vi "Dialog_Configure Tiling.vi"(9 "Index of Tiling":i32, 10 "Tbl Refnum":refnum<vi>, 11 "Tree Refnum":refnum<vi>) -> (1 "Empty Array/Cancelled?":bool, 2 "Index of 2DFrame.Scan":i32, 3 "Updated Macro String Array":string[](array[string]), 4 "Skip configure 2D settings?":bool)   [LabVIEW 2012]
doc: "SciScan 1.2 160622"
uses:
  Z-Scan Types.ctl
  Custom Controls/scan mode main settings tab.ctl
  FGV_MacroCore_Commands.ctl
  Create Preset commands ENUM.ctl
  GFG/GFGnumericGet.vi
  GFG/GFGfpRefGet.vi
  GFG/GFG library.lvlib
panel:
  out "bottom/right abs":cluster{"abs x":dbl, "abs y":dbl, "abs z":dbl}
  out "bottom/right rel":cluster{"rel x":dbl, "rel y":dbl, "rel z":dbl}
  out "top/left rel":cluster{"rel x":dbl, "rel y":dbl, "rel z":dbl}
  out "top/left abs":cluster{"abs x":dbl, "abs y":dbl, "abs z":dbl}
  in  "Add Bottom/Right Pos":bool
  in  "Add Top/Left Pos":bool
  in  "Cancel Button":bool
  in  "Tiling Type":T1=enum."Slow Z"
  in  "Overlap %":dbl=20.0 min=-100.0 max=100.0
  in  "Frames Per Tile":dbl caption="Frames/Tile" min=4.0 step=4.0
  in  "OK Button":bool
  out "error out":errorcluster
  in  "error in (no error)":errorcluster
  # "You have selected the Tiling Preset \nThe Macro for carrying out the Tiling will be auto-generated for you\nbased on your configuration"
  # "Please note that stitching of tiled images is not supported"
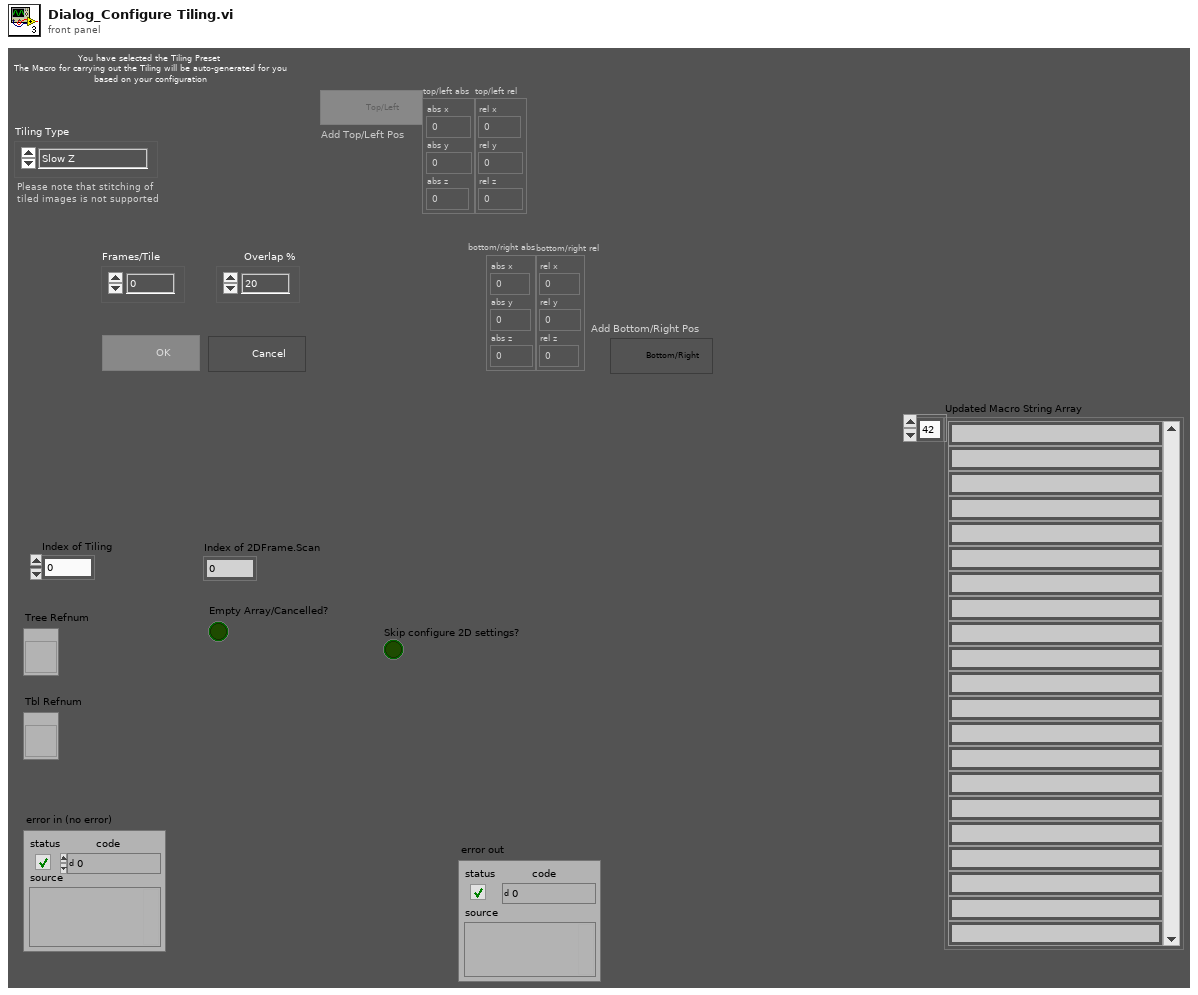
[diagram p1: front panel]
types:
  T1 = typedef "Z-Scan Types.ctl" = enum16{"Single Plane", "Slow Z", "Z-Stack (Regular)", "Fast Z (Piezo)"}
  T2 = typedef "scan mode main settings tab.ctl" = enum32{"2D frame", "2D line scan", "general settings", "Z Stack", "piezo"}
  T3 = cluster{"OK Button":refnum<vi>, "Add Top/Left Pos":refnum<vi>, "Add Bottom/Right Pos":refnum<vi>}
  T4 = enum8{"Enabled", "Disabled", "Disabled and Grayed Out"}
  T5 = typedef "FGV_MacroCore_Commands.ctl" = enum16{"Initialize", "Get Array", "Load macro from file", "Insert Item", "Insert at End", "Edit Parameter String", "Delete instruction", "Move Items", "Save", "SaveAs", "UpdateInfoTable", "Edit Settings File", "New Macro", "Read Temp File", "Delete Multiple"}
  T6 = cluster{"Left Cell String":string, "Child Text":string[], "Child Tag":string, "Item Indent":i32, "Child Only?":bool, "Glyph Index":i32}
  T7 = typedef "Create Preset commands ENUM.ctl" = enum16{"Slow.Z_Move.To.Pos", "Slow.Z_Laser.Power", "Slow.Z_Record", "Tiling_Move.To.Pos", "Tiling_Laser.Power", "Tiling_Record"}
  T8 = cluster{"Left Cell String":string, "Child Text":string[], "Child Tag":string, "Item Indent":i32, "Child Only?":bool, "Glyph Index":i32}[]
  T9 = cluster{"WaveformChartRef":refnum<vi>, "DigitalRef":refnum<vi>, "ArrayRef":refnum<vi>, "TabControlRef":refnum<vi>, "EnumRef":refnum<vi>, "RingRef":refnum<vi>, "BooleanRef":refnum<vi>, "KnobRef":refnum<vi>, "SlideRef":refnum<vi>, "PathRef":refnum<vi>, "StringRef":refnum<vi>, "ComboBox":refnum<vi>, "WaveformGraphRef":refnum<vi>}
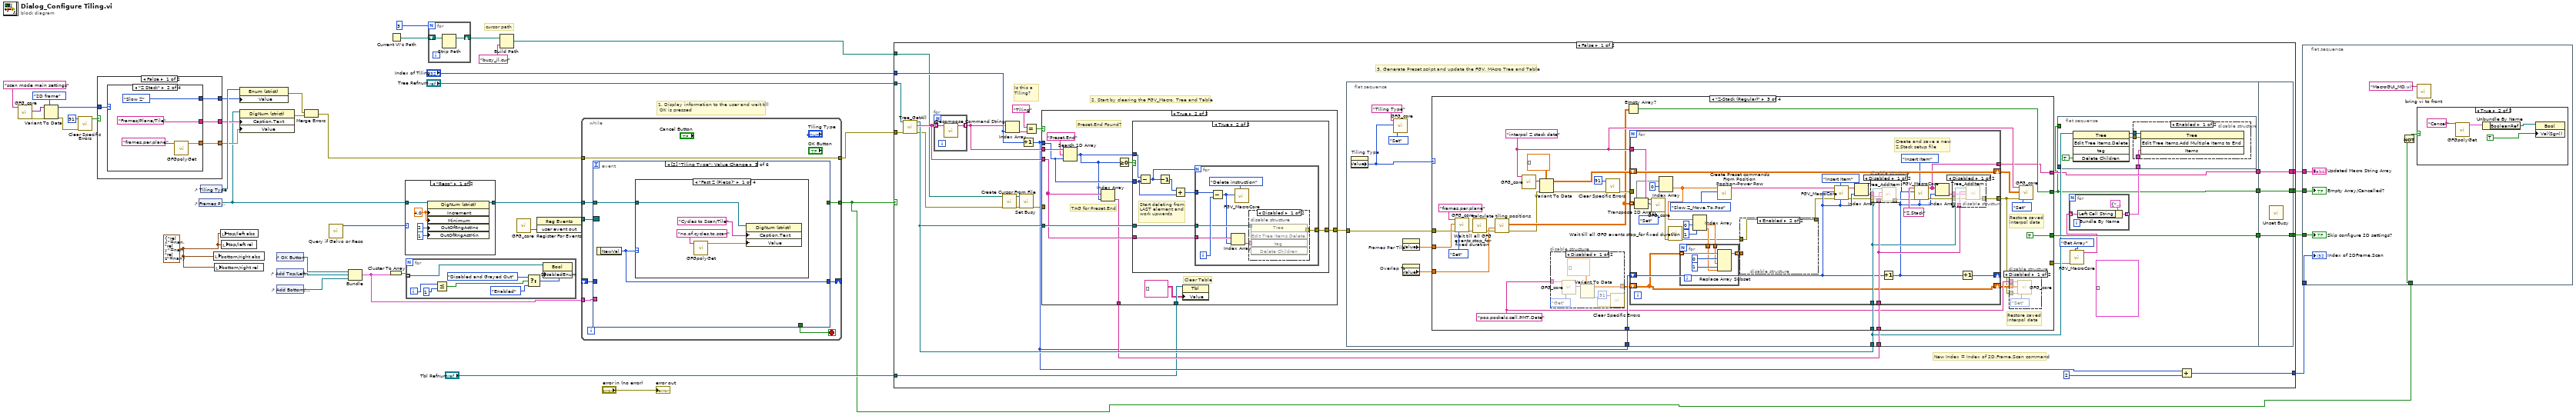
[diagram p0: block diagram]
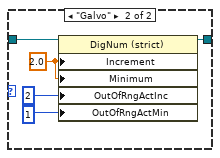
[diagram p3: hidden frame]
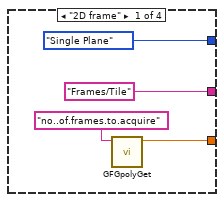
[diagram p4: hidden frame]
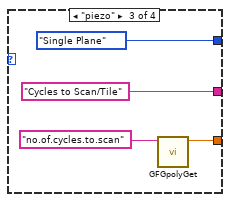
[diagram p5: hidden frame]
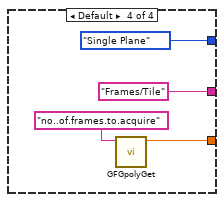
[diagram p6: hidden frame]
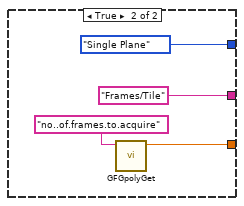
[diagram p7: hidden frame]
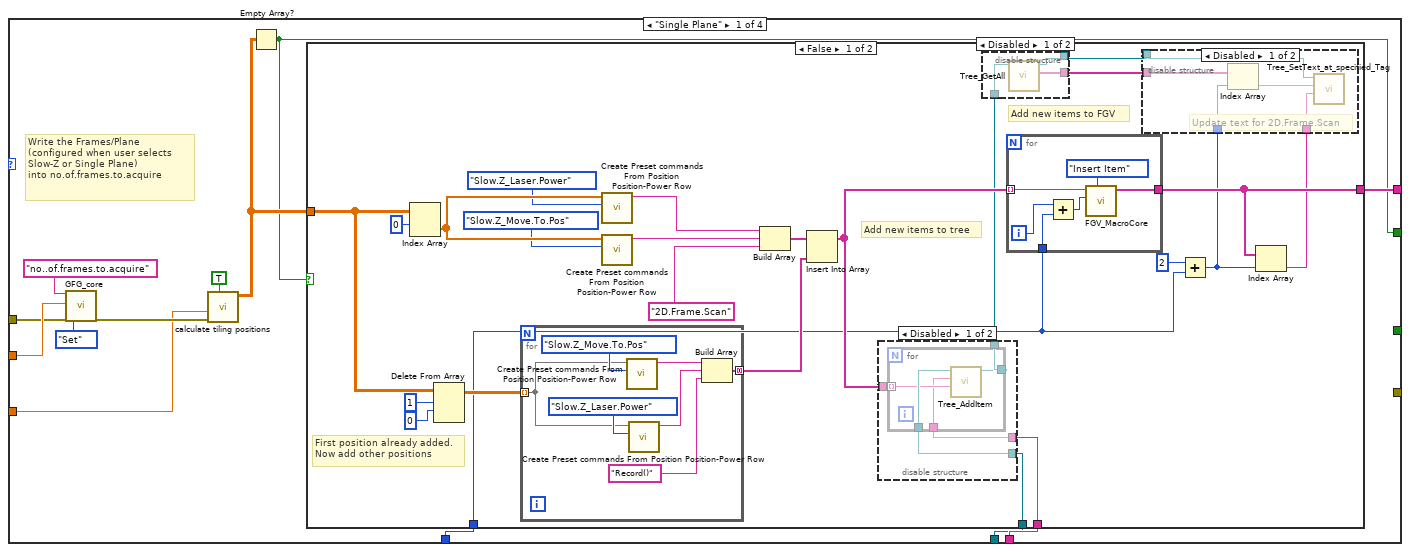
[diagram p9: hidden frame]
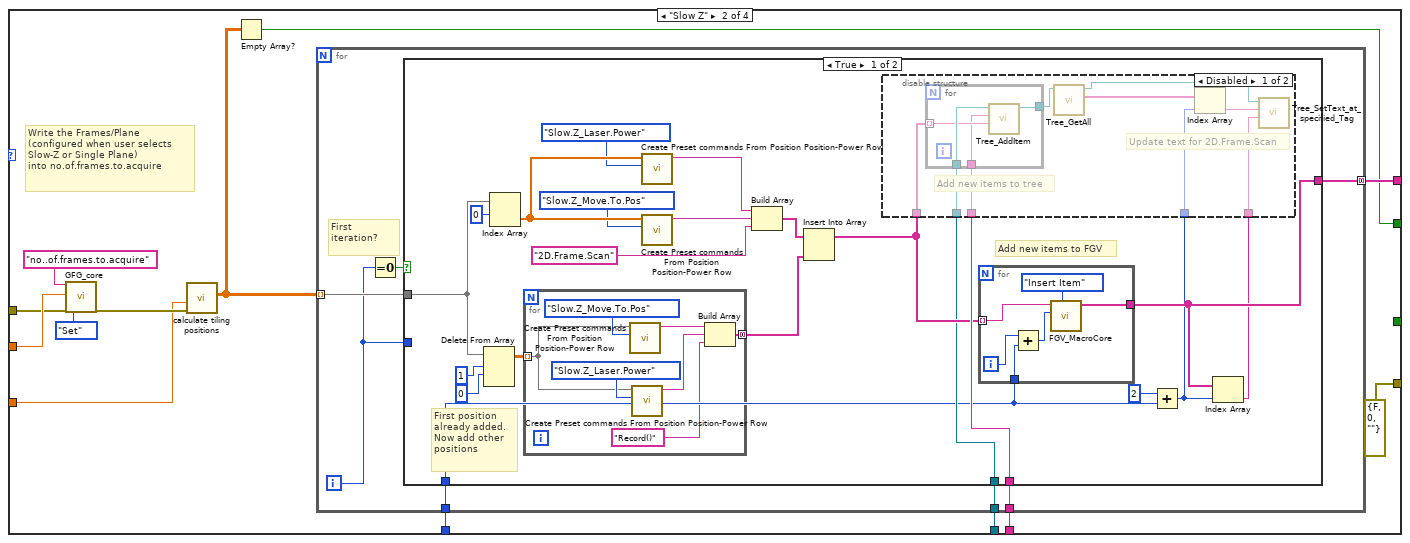
[diagram p14: hidden frame]
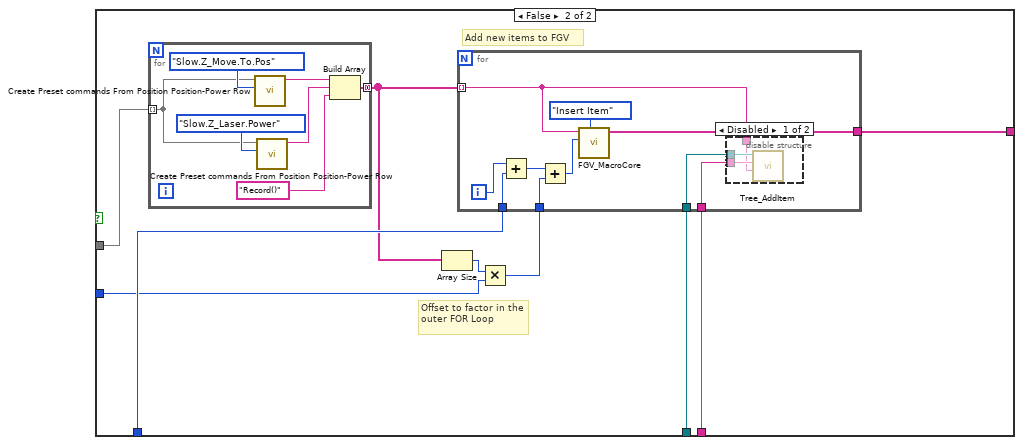
[diagram p16: hidden frame]
diagram:
  w1 = cluster{"rel x":dbl, "rel y":dbl, "rel z":dbl} {"rel x"=nan, "rel y"=nan, "rel z"=nan} ("rel pos out")
  # "1. Display information to the user and wait till\n OK is pressed"
  # "cursor path"
  n1 = call "GFG_core.vi"("Variable Name in"="scan mode main settings") -> ("Variant Out"=w23:variant, "error out"=w22:errorcluster)  [unwired: 12 in, 5 out]
  n2 = Variant To Data(error in=w22, type=scan_mode_main_settings_tab."2D frame" ("scan mode main settings"), Variant=w23) -> (data=w18:T2, error out=w20:errorcluster)
  n3 = call "Clear Specific Errors.vi"("Error In"=w20, "Error number In"=91) -> ("Error Cleared?"=w19:bool)  [unwired: 8 in, 1 out]
  n4 = case shown="False" w19 {
    tunnel: w18 -> [w45 _]
    tunnel: [w44 Z-Scan_Types."Single Plane" ("Value")] -> w16
    tunnel: [w43 "Frames/Tile" ("Caption.Text")] -> w15
    tunnel: [w42 w62] -> w14
    frame False {
      n5 = case shown="\"Z Stack\"" w45 {
        tunnel: [Z-Scan_Types."Single Plane" ("Value") Z-Scan_Types."Slow Z" ("Value") Z-Scan_Types."Single Plane" ("Value") Z-Scan_Types."Single Plane" ("Value")] -> w44
        tunnel: ["Frames/Tile" ("Caption.Text") "Frames/Plane/Tile" ("Caption.Text") "Cycles to Scan/Tile" ("Caption.Text") "Frames/Tile" ("Caption.Text")] -> w43
        tunnel: [w46 w52 w56 w58] -> w42
        frame "2D frame" {
          n6 = call-poly "GFGpolyGet.vi"("Variable Name in"="no..of.frames.to.acquire") -> ("Numeric"=w46:dbl)  [unwired: 8 in, 2 out]
        }
        frame "Z Stack" {
          n7 = call-poly "GFGpolyGet.vi"("Variable Name in"="frames.per.plane") -> ("Numeric"=w52:dbl)  [unwired: 8 in, 2 out]
        }
        frame "piezo" {
          n8 = call-poly "GFGpolyGet.vi"("Variable Name in"="no.of.cycles.to.scan") -> ("Numeric"=w56:dbl)  [unwired: 8 in, 2 out]
        }
        frame Default {
          n9 = call-poly "GFGpolyGet.vi"("Variable Name in"="no..of.frames.to.acquire") -> ("Numeric"=w58:dbl)  [unwired: 8 in, 2 out]
        }
      }
    }
    frame True {
      n10 = call-poly "GFGpolyGet.vi"("Variable Name in"="no..of.frames.to.acquire") -> ("Numeric"=w62:dbl)  [unwired: 8 in, 2 out]
    }
  }
  n11 = control-ref of="Frames Per Tile"() -> (w9:refnum<vi>)
  n12 = control-ref of="Tiling Type"() -> (w17:refnum<vi>)
  n13 = local write "bottom/right abs"(w1) -> ()
  n14 = local write "bottom/right rel"(w1) -> ()
  n15 = local write "top/left abs"(w1) -> ()
  n16 = local write "top/left rel"(w1) -> ()
  n17 = property class="Enum (strict)"(reference=w17, "Value"=w16) -> (error out=w13:errorcluster)  [unwired: 1 in, 1 out]
  n18 = property class="DigNum (strict)"(reference=w9, "Caption.Text"=w15, "Value"=w14) -> (error out=w12:errorcluster)  [unwired: 1 in, 1 out]
  n19 = control-ref of="OK Button"() -> (w7:refnum<vi>)
  n20 = control-ref of="Add Top/Left Pos"() -> (w6:refnum<vi>)
  n21 = control-ref of="Add Bottom/Right Pos"() -> (w5:refnum<vi>)
  n22 = Merge Errors(w13, w12) -> (w11:errorcluster)
  n23 = call "Query if Galvo or Reso.vi"() -> ("System Type"=w10:enum16{"Galvo", "Reso"})  [unwired: 10 in, 1 out]
  n24 = Bundle("OK Button"=w7, "Add Top/Left Pos"=w6, "Add Bottom/Right Pos"=w5) -> (w3:T3)  [unwired: 1 in]
  n25 = Cluster To Array(cluster=w3) -> (array=w4:refnum<vi>[])
  n26 = Current VI's Path() -> (path=w35:path)
  n27 = case shown="\"Reso\"" w10 {
    tunnel: w9 -> [w70 w75]
    tunnel: [w67 w72] -> w8
    frame "Reso" {
      w69 = 4.0 ("Data Entry Limits:Increment")
      n28 = property class="DigNum (strict)"(reference=w70, "Increment"=w69, "Minimum"=w69, "OutOfRngActInc"=u8 2 ("Response to Value Outside Limits:Minimum"), "OutOfRngActMin"=u8 1 ("Response to Value Outside Limits:Minimum")) -> (reference out=w67:refnum<vi>)  [unwired: 1 in, 1 out]
    }
    frame "Galvo" {
      w74 = 2.0 ("Data Entry Limits:Increment")
      n29 = property class="DigNum (strict)"(reference=w75, "Increment"=w74, "Minimum"=w74, "OutOfRngActInc"=u8 2 ("Response to Value Outside Limits:Minimum"), "OutOfRngActMin"=u8 1 ("Response to Value Outside Limits:Minimum")) -> (reference out=w72:refnum<vi>)  [unwired: 1 in, 1 out]
    }
  }
  n30 = for {
    tunnel: w4 -> [w82] mode=indexing
    i -> [w81]
    n31 = Less Or Equal?(x=w81, y=1) -> (x <= y?=w77:bool)
    n32 = Select(t=T4."Disabled and Grayed Out" ("Disabled"), s=w77, f=T4."Enabled" ("Disabled")) -> (s? t:f=w76:T4)
    n33 = property class="Bool"(reference=w82, "DisabledEnum"=w76) -> ()  [unwired: 1 in, 2 out]
  }
  n34 = for {
    N: 3 -> [_]
    shift-right: [w83] -> w34
    shift-left: w35 -> [w84]
    n35 = Strip Path(path=w84) -> (stripped path=w83:path)  [unwired: 1 out]
  }
  n36 = Build Path(base path=w34, name or relative path="busy_il.cur") -> (appended path=w28:path)
  n37 = call "GFG_core.vi"() -> ("user event out"=w41:refnum<user-event>)  [unwired: 13 in, 6 out]
  n38 = register-events(w41) -> (reference out=w40:refnum<event-registration>)  [unwired: 2 in, 1 out]
  n39 = while {
    tunnel: w40 -> [w92]
    tunnel: w11 -> [w90]
    tunnel: [w90] -> w26
    tunnel: [w89] -> w2
    tunnel: w8 -> [w88]
    shift-right: [w87] -> _
    shift-left: _ -> [w86]
    tunnel: w3 -> [w85]
    stop <- w91 stop-if-true
    n40 = event shown="[2] \"Tiling Type\": Value Change" {
      selector: w92 -> [_ _ _ _ _ _]
      dyn-events: _ -> [_ _ _ _ _ _]
      timeout: _ -> [_ _ _ _ _ _]
      tunnel: [TRUE w102 _ _ _ w142] -> w91
      tunnel: [_ _ _ _ _ w142] -> w89
      tunnel: w88 -> [_ _ w106 _ _ _]
      tunnel: [w99 w101 w105 w132 w140 w141] -> w87
      tunnel: w86 -> [w99 w101 _ w132 w140 w141]
      tunnel: w85 -> [_ _ _ w127 w134 _]
      event "OK Button": Value Change {
        n41 = event-data() -> ()  [unwired: 1 in, 1 out]
        n42 = call "GFG_core.vi"("Variable Name in"="Frames Per Tile", "Variant in"="Frames Per Tile", "Action"=enum16{"Init", "Set", "Get", "Clear"}."Set") -> ()  [unwired: 10 in, 7 out]
        n43 = call "GFG_core.vi"("Variable Name in"="Overlap", "Variant in"="Overlap %", "Action"=enum16{"Init", "Set", "Get", "Clear"}."Set") -> ()  [unwired: 10 in, 7 out]
      }
      event User Event {
        n44 = event-data() -> ("Variable Name"=w103:string)  [unwired: 1 in]
        n45 = case shown="\"QUIT\"" w103 {
          tunnel: [_ TRUE] -> w102
          frame "False", Default {
          }
          frame "QUIT" {
          }
        }
      }
      event Value Change {
        n46 = event-data() -> ("NewVal"=w105:T1)  [unwired: 1 in]
        n47 = case shown="\"Fast Z (Piezo)\"" w105 {
          tunnel: w106 -> [w108 w112 w117 w121]
          frame "Fast Z (Piezo)" {
            n48 = call-poly "GFGpolyGet.vi"("Variable Name in"="no.of.cycles.to.scan") -> ("Numeric"=w107:dbl)  [unwired: 8 in, 2 out]
            n49 = property class="DigNum (strict)"(reference=w108, "Caption.Text"="Cycles to Scan/Tile", "Value"=w107) -> ()  [unwired: 1 in, 2 out]
          }
          frame "Slow Z" {
            n50 = call-poly "GFGpolyGet.vi"("Variable Name in"="frames.per.plane") -> ("Numeric"=w111:dbl)  [unwired: 8 in, 2 out]
            n51 = property class="DigNum (strict)"(reference=w112, "Caption.Text"="Frames/Plane/Tile", "Value"=w111) -> ()  [unwired: 1 in, 2 out]
          }
          frame "Z-Stack (Regular)" {
            n52 = call-poly "GFGpolyGet.vi"("Variable Name in"="frames.per.plane") -> ("Numeric"=w116:dbl)  [unwired: 8 in, 2 out]
            n53 = property class="DigNum (strict)"(reference=w117, "Caption.Text"="Frames/Plane/Tile", "Value"=w116) -> ()  [unwired: 1 in, 2 out]
          }
          frame "Single Plane" {
            n54 = call-poly "GFGpolyGet.vi"("Variable Name in"="no..of.frames.to.acquire") -> ("Numeric"=w119:dbl)  [unwired: 8 in, 2 out]
            n55 = property class="DigNum (strict)"(reference=w121, "Caption.Text"="Frames/Tile", "Value"=w119) -> ()  [unwired: 1 in, 2 out]
          }
        }
      }
      event "Add Top/Left Pos": Value Change {
        n56 = event-data() -> ()  [unwired: 1 in, 1 out]
        n57 = Unbundle By Name(w127) -> ("Add Bottom/Right Pos"=w125:refnum<vi>, "OK Button"=w123:refnum<vi>)
        n58 = call "current abs pos to rel pos.vi"() -> ("rel pos out"=w128:cluster{"rel x":dbl, "rel y":dbl, "rel z":dbl}, "abs pos out"=→"top/left abs":cluster{"abs x":dbl, "abs y":dbl, "abs z":dbl})  [unwired: 10 in]
        "top/left rel" <- w128
        n59 = property class="Bool"(reference=w125, "DisabledEnum"=T4."Disabled and Grayed Out" ("Disabled")) -> ()  [unwired: 1 in, 2 out]
        n60 = property class="Bool"(reference=w123, "DisabledEnum"=T4."Enabled" ("Disabled")) -> ()  [unwired: 1 in, 2 out]
        n61 = call "GFG_core.vi"("Variable Name in"="top left tile pos", "Variant in"=w128, "Action"=enum16{"Init", "Set", "Get", "Clear"}."Set") -> ()  [unwired: 10 in, 7 out]
      }
      event "Add Bottom/Right Pos": Value Change {
        n62 = event-data() -> ()  [unwired: 1 in, 1 out]
        n63 = Unbundle By Name(w134) -> ("Add Top/Left Pos"=w133:refnum<vi>)
        n64 = call "current abs pos to rel pos.vi"() -> ("rel pos out"=w137:cluster{"rel x":dbl, "rel y":dbl, "rel z":dbl}, "abs pos out"=→"bottom/right abs":cluster{"abs x":dbl, "abs y":dbl, "abs z":dbl})  [unwired: 10 in]
        "bottom/right rel" <- w137
        n65 = property class="Bool"(reference=w133, "DisabledEnum"=T4."Enabled" ("Disabled")) -> ()  [unwired: 1 in, 2 out]
        n66 = call "GFG_core.vi"("Variable Name in"="bottom right tile pos", "Variant in"=w137, "Action"=enum16{"Init", "Set", "Get", "Clear"}."Set") -> ()  [unwired: 10 in, 7 out]
      }
      event "Cancel Button": Value Change {
        w142 = TRUE
        n67 = event-data() -> ()  [unwired: 1 in, 1 out]
      }
    }
  }
  n68 = case shown="False" w2 {
    selector: w2 -> [_ w577]
    tunnel: "Index of Tiling" -> [w162 _]
    tunnel: "Tree Refnum" -> [w161 _]
    tunnel: [w159 _] -> w36
    tunnel: "Tbl Refnum" -> [w153 _]
    tunnel: [w152 _] -> w30
    tunnel: [w151 w577] -> w29
    tunnel: w28 -> [w148 _]
    tunnel: [w145 _] -> w27
    tunnel: w26 -> [w144 _]
    frame False {
      # "New Index = Index of 2D.Frame.Scan command"
      # "3. Generate Preset script and update the FGV, MAcro Tree and Table"
      # "2. Start by clearing the FGV_Macro, Tree and Table"
      # "Is this a Tiling?"
      n69 = call "Tree_GetAll.vi"("Error In"=w144, "Tree Refnum IN"=w161) -> ("Error Out"=w147:errorcluster, "Tags"=w158:string[], "Tree Refnum OUT"=w156:refnum<vi>)  [unwired: 6 in, 1 out]
      n70 = for {
        tunnel: w158 -> [w546] mode=indexing
        tunnel: [w545] -> w157 mode=indexing
        n71 = call "Decompose Command String.vi"("Command IN"=w546) -> ("Action"=w545:string)  [unwired: 7 in, 3 out]
      }
      n72 = call <vilib>:"Create Cursor From File.vi"("error in (no error)"=w147, "cursor file"=w148) -> ("error out"=w150:errorcluster, "cursor ID"=w149:refnum<k1>)  [unwired: 8 in]
      n73 = Index Array(array=w157, index=w162) -> (element=w165:string)
      n74 = call <vilib>:"Set Busy.vi"("error in (no error)"=w150, "cursor ID"=w149) -> ("error out"=w146:errorcluster)  [unwired: 8 in, 1 out]
      n75 = Increment(x=w162) -> (x+1=w154:i32)
      n76 = Equal?(x="Tiling" ("Variable Name in"), y=w165) -> (x = y?=w163:bool)
      n77 = case shown="True" w163 {
        tunnel: w158 -> [_ w553]
        tunnel: w157 -> [_ w557]
        tunnel: w154 -> [_ w551]
        tunnel: w156 -> [_ w555]
        tunnel: [_ w554] -> w143
        tunnel: [_ w550] -> w155
        tunnel: w153 -> [_ w548]
        tunnel: w146 -> [_ _]
        frame False {
        }
        frame True {
          # "Clear Table"
          # "TAG for Preset.End"
          # "Preset.End Found?"
          n78 = Search 1D Array(1D array=w557, element="Preset.End", start index (0)=w551) -> (index of element=w549:i32)
          n79 = Index Array(array=w553, index=w549) -> (element=w550:string)
          n80 = Greater Or Equal To 0?(x=w549) -> (x >= 0?=w552:bool)
          n81 = case shown="True" w552 {
            tunnel: w549 -> [_ w565]
            tunnel: w555 -> [_ w561]
            tunnel: [_ w560] -> w554
            tunnel: w551 -> [_ w559]
            tunnel: w553 -> [_ w558]
            frame False {
            }
            frame True {
              # "Start deleting from LAST element and work upwards"
              n82 = Subtract(x=w565, y=w559) -> (x-y=w564:i32)
              n83 = Decrement(x=w564) -> (x-1=w563:i32)
              n84 = Add(x=w563, y=w559) -> (x+y=w562:i32)
              n85 = for {
                N: w564 -> [_]
                tunnel: w562 -> [w571]
                tunnel: w561 -> [w570]
                tunnel: w558 -> [w569]
                tunnel: [w566] -> w560
                i -> [w572]
                n86 = Subtract(x=w571, y=w572) -> (x-y=w568:i32)
                n87 = Index Array(array=w569, index=w568) -> (element=w567:string)
                n88 = call "FGV_MacroCore.vi"("MacroFGV_Commands"=FGV_MacroCore_Commands."Delete instruction", "Start Index"=w568) -> ()  [unwired: 5 in, 5 out]
                n89 = disable-structure shown="Disabled" {
                  disable-tunnel: w570 -> [w576 _]
                  disable-tunnel: w567 -> [w575 _]
                  disable-tunnel: [w574 _] -> w566
                  frame Disabled {
                    n90 = invoke class="Tree" method="Edit Tree Items.Delete"(reference=w576, "tag"=w575) -> (error out=w574:errorcluster)  [unwired: 3 in, 4 out]
                  }
                  frame Enabled {
                  }
                }
              }
            }
          }
          n91 = property class="Tbl"(reference=w548, "Value"=string[][] []) -> ()  [unwired: 1 in, 2 out]
        }
      }
      n92 = flat-sequence {
        tunnel: w156 -> [w178]
        tunnel: w155 -> [w184]
        tunnel: w154 -> [w183]
        tunnel: [w177] -> w168
        tunnel: [w175] -> w167
        tunnel: [w181] -> w166
        tunnel: w143 -> [w182]
        tunnel: [w543] -> w151
        tunnel: [w544] -> w152
        tunnel: w168 -> [w544]
        tunnel: w167 -> [w543]
        tunnel: [w542] -> w145
        tunnel: w166 -> [w542]
        frame #0 {
          (unwired) T8 [] ("Items")
          n93 = property on="Tiling Type" class="Enum (strict)"() -> ("Value"=w169:T1)  [unwired: 2 in, 2 out]
          n94 = call "GFG_core.vi"("Variable Name in"="Tiling Type", "Variant in"=w169, "Action"=enum16{"Init", "Set", "Get", "Clear"}."Set") -> ()  [unwired: 10 in, 7 out]
          n95 = property on="Frames Per Tile" class="DigNum (strict)"() -> ("Value"=w180:dbl)  [unwired: 2 in, 2 out]
          n96 = property on="Overlap %" class="DigNum (strict)"() -> ("Value"=w179:dbl)  [unwired: 2 in, 2 out]
          n97 = case shown="\"Z-Stack (Regular)\"" w169 {
            tunnel: w178 -> [w207 w273 w373 w477]
            tunnel: w184 -> [w208 w274 w372 w476]
            tunnel: w183 -> [w206 w272 w377 w481]
            tunnel: [w205 w271 w371 w475] -> w177
            tunnel: [w196 w264 w384 w488] -> w175
            tunnel: w182 -> [w201 w267 w365 w460]
            tunnel: [_ _ TRUE TRUE] -> w181
            tunnel: w180 -> [w204 w270 w361 w459]
            tunnel: w179 -> [w199 w265 w358 w457]
            tunnel: [_ errorcluster {"status"=FALSE, "code"=0, "source"=""} ("error in (no error)") _ _] -> w172
            frame "Single Plane" {
              # "Write the Frames/Plane\n(configured when user selects Slow-Z or Single Plane)\ninto no.of.frames.to.acquire"
              n98 = call "GFG_core.vi"("Variable Name in"="no..of.frames.to.acquire", "Variant in"=w204, "error in (no error)"=w201, "Action"=enum16{"Init", "Set", "Get", "Clear"}."Set") -> ("error out"=w200:errorcluster)  [unwired: 9 in, 6 out]
              n99 = call "calculate tiling positions.vi"("Single Plane?"=TRUE, "error in (no error)"=w200, "overlap percentage"=w199) -> ("2D Array for single plane tiling or Slow Z Tiling"=w198:dbl[][])  [unwired: 6 in, 2 out]
              n100 = Empty Array?(array=w198) -> (empty?=w196:bool)
              n101 = case shown="False" w196 {
                tunnel: w208 -> [w222 _]
                tunnel: w207 -> [w218 _]
                tunnel: w206 -> [w216 _]
                tunnel: [w214 _] -> w205
                tunnel: w198 -> [w209 _]
                frame False {
                  # "Add new items to FGV"
                  # "Add new items to tree"
                  # "First position already added.\nNow add other positions"
                  n102 = Index Array(array=w209, index (row)=0) -> (element=w225:dbl[])  [unwired: 1 in]
                  n103 = Delete From Array(array=w209, length=1, index (row)=0) -> (array with subset deleted=w230:dbl[][])  [unwired: 1 in, 1 out]
                  n104 = for {
                    tunnel: w230 -> [w252] mode=indexing
                    tunnel: [w255] -> w227 mode=concatenating
                    n105 = call "Create Preset commands From Position Position-Power Row.vi"("Create SlowZ commands_Enum"=Create_Preset_commands_ENUM."Slow.Z_Move.To.Pos", "Position-Power Row"=w252) -> ("concatenated string"=w251:string)  [unwired: 9 in]
                    n106 = call "Create Preset commands From Position Position-Power Row.vi"("Create SlowZ commands_Enum"=Create_Preset_commands_ENUM."Slow.Z_Laser.Power", "Position-Power Row"=w252) -> ("concatenated string"=w250:string)  [unwired: 9 in]
                    n107 = Build Array(w251, w250, "Record()" ("Variable Name in")) -> (w255:string[])
                  }
                  n108 = call "Create Preset commands From Position Position-Power Row.vi"("Create SlowZ commands_Enum"=Create_Preset_commands_ENUM."Slow.Z_Laser.Power", "Position-Power Row"=w225) -> ("concatenated string"=w219:string)  [unwired: 9 in]
                  n109 = call "Create Preset commands From Position Position-Power Row.vi"("Create SlowZ commands_Enum"=Create_Preset_commands_ENUM."Slow.Z_Move.To.Pos", "Position-Power Row"=w225) -> ("concatenated string"=w220:string)  [unwired: 9 in]
                  n110 = Build Array(w219, w220, "2D.Frame.Scan" ("Variable Name in")) -> (w228:string[])
                  n111 = Insert Into Array(array=w228, new element=w227) -> (w221:string[])  [unwired: 1 in]
                  n112 = disable-structure shown="Disabled" {
                    disable-tunnel: w222 -> [w239 _]
                    disable-tunnel: w221 -> [w238 _]
                    disable-tunnel: w218 -> [w237 _]
                    disable-tunnel: [w236 _] -> w217
                    frame Disabled {
                      n113 = for {
                        tunnel: w238 -> [w242] mode=indexing
                        tunnel: w237 -> [w243]
                        tunnel: w239 -> [w241]
                        tunnel: [w240] -> w236
                        n114 = call "Tree_AddItem.vi"("NEW String"=w242, "Tag at add position"=w241, "Tree Refnum"=w243) -> ("Tree Refnum OUT"=w240:refnum<vi>)  [unwired: 6 in, 2 out]
                      }
                    }
                    frame Enabled {
                    }
                  }
                  n115 = disable-structure shown="Disabled" {
                    disable-tunnel: w217 -> [w235 _]
                    disable-tunnel: [w234 _] -> w213
                    disable-tunnel: [w233 _] -> w211
                    frame Disabled {
                      n116 = call "Tree_GetAll.vi"("Tree Refnum IN"=w235) -> ("Tags"=w234:string[], "Tree Refnum OUT"=w233:refnum<vi>)  [unwired: 7 in, 2 out]
                    }
                    frame Enabled {
                    }
                  }
                  n117 = for {
                    tunnel: w221 -> [w248] mode=indexing
                    tunnel: [w245] -> w214
                    tunnel: w216 -> [w246]
                    i -> [w247]
                    n118 = Add(x=w247, y=w246) -> (x+y=w244:i32)
                    n119 = call "FGV_MacroCore.vi"("MacroFGV_Commands"=FGV_MacroCore_Commands."Insert Item", "Start Index"=w244, "Macro Command or Info (String)"=w248) -> ("Macro String Array"=w245:string[])  [unwired: 4 in, 4 out]
                  }
                  n120 = Add(x=2 ("y"), y=w216) -> (x+y=w212:i32)
                  n121 = Index Array(array=w214, index=w212) -> (element=w210:string)
                  n122 = disable-structure shown="Disabled" {
                    disable-tunnel: w213 -> [w261 _]
                    disable-tunnel: w212 -> [w260 _]
                    disable-tunnel: w211 -> [w258 _]
                    disable-tunnel: w210 -> [w257 _]
                    frame Disabled {
                      # "Update text for 2D.Frame.Scan"
                      n123 = Index Array(array=w261, index=w260) -> (element=w259:string)
                      n124 = call "Tree_SetText_at_specified_Tag.vi"("New String IN"=w257, "Tag (whose string to be edited)"=w259, "Tree Refnum IN"=w258) -> ()  [unwired: 7 in, 2 out]
                    }
                    frame Enabled {
                    }
                  }
                }
                frame True {
                }
              }
            }
            frame "Slow Z" {
              # "Write the Frames/Plane\n(configured when user selects Slow-Z or Single Plane)\ninto no.of.frames.to.acquire"
              n125 = call "GFG_core.vi"("Variable Name in"="no..of.frames.to.acquire", "Variant in"=w270, "error in (no error)"=w267, "Action"=enum16{"Init", "Set", "Get", "Clear"}."Set") -> ("error out"=w266:errorcluster)  [unwired: 9 in, 6 out]
              n126 = call "calculate tiling positions.vi"("error in (no error)"=w266, "overlap percentage"=w265) -> ("Array 2 - for Zstack tiling use this"=w263:dbl[][][])  [unwired: 7 in, 2 out]
              n127 = Empty Array?(array=w263) -> (empty?=w264:bool)
              n128 = for {
                tunnel: w274 -> [w281]
                tunnel: w273 -> [w280]
                tunnel: w272 -> [w279]
                tunnel: [w278] -> w271 mode=concatenating
                tunnel: w263 -> [w277] mode=indexing
                i -> [w275]
                # "First iteration?"
                n129 = Equal To 0?(x=w275) -> (x = 0?=w276:bool)
                n130 = case shown="True" w276 {
                  tunnel: w281 -> [w293 w330]
                  tunnel: w280 -> [w289 w329]
                  tunnel: w279 -> [w288 w337]
                  tunnel: [w286 w336] -> w278
                  tunnel: w277 -> [w283 w335]
                  tunnel: w275 -> [_ w332]
                  frame True {
                    # "Add new items to FGV"
                    # "First position already added. Now add other positions"
                    n131 = Delete From Array(array=w283, length=1, index (row)=0) -> (array with subset deleted=w300:dbl[][])  [unwired: 1 in, 1 out]
                    n132 = Index Array(array=w283, index (row)=0) -> (element=w296:dbl[])  [unwired: 1 in]
                    n133 = for {
                      tunnel: w300 -> [w324] mode=indexing
                      tunnel: [w327] -> w298 mode=concatenating
                      n134 = call "Create Preset commands From Position Position-Power Row.vi"("Create SlowZ commands_Enum"=Create_Preset_commands_ENUM."Slow.Z_Move.To.Pos", "Position-Power Row"=w324) -> ("concatenated string"=w323:string)  [unwired: 9 in]
                      n135 = call "Create Preset commands From Position Position-Power Row.vi"("Create SlowZ commands_Enum"=Create_Preset_commands_ENUM."Slow.Z_Laser.Power", "Position-Power Row"=w324) -> ("concatenated string"=w322:string)  [unwired: 9 in]
                      n136 = Build Array(w323, w322, "Record()" ("Variable Name in")) -> (w327:string[])
                    }
                    n137 = call "Create Preset commands From Position Position-Power Row.vi"("Create SlowZ commands_Enum"=Create_Preset_commands_ENUM."Slow.Z_Laser.Power", "Position-Power Row"=w296) -> ("concatenated string"=w290:string)  [unwired: 9 in]
                    n138 = call "Create Preset commands From Position Position-Power Row.vi"("Create SlowZ commands_Enum"=Create_Preset_commands_ENUM."Slow.Z_Move.To.Pos", "Position-Power Row"=w296) -> ("concatenated string"=w291:string)  [unwired: 9 in]
                    n139 = Build Array(w290, w291, "2D.Frame.Scan" ("Variable Name in")) -> (w299:string[])
                    n140 = Insert Into Array(array=w299, new element=w298) -> (w292:string[])  [unwired: 1 in]
                    n141 = for {
                      tunnel: w292 -> [w320] mode=indexing
                      tunnel: [w317] -> w286
                      tunnel: w288 -> [w318]
                      i -> [w319]
                      n142 = Add(x=w319, y=w318) -> (x+y=w316:i32)
                      n143 = call "FGV_MacroCore.vi"("MacroFGV_Commands"=FGV_MacroCore_Commands."Insert Item", "Start Index"=w316, "Macro Command or Info (String)"=w320) -> ("Macro String Array"=w317:string[])  [unwired: 4 in, 4 out]
                    }
                    n144 = Add(x=2 ("y"), y=w288) -> (x+y=w285:i32)
                    n145 = Index Array(array=w286, index=w285) -> (element=w284:string)
                    n146 = disable-structure shown="Disabled" {
                      disable-tunnel: w293 -> [w311 _]
                      disable-tunnel: w292 -> [w310 _]
                      disable-tunnel: w289 -> [w309 _]
                      disable-tunnel: w285 -> [w306 _]
                      disable-tunnel: w284 -> [w303 _]
                      frame Disabled {
                        # "Update text for 2D.Frame.Scan"
                        # "Add new items to tree"
                        n147 = for {
                          tunnel: w310 -> [w314] mode=indexing
                          tunnel: w309 -> [w315]
                          tunnel: w311 -> [w313]
                          tunnel: [w312] -> w308
                          n148 = call "Tree_AddItem.vi"("NEW String"=w314, "Tag at add position"=w313, "Tree Refnum"=w315) -> ("Tree Refnum OUT"=w312:refnum<vi>)  [unwired: 6 in, 2 out]
                        }
                        n149 = call "Tree_GetAll.vi"("Tree Refnum IN"=w308) -> ("Tags"=w307:string[], "Tree Refnum OUT"=w304:refnum<vi>)  [unwired: 7 in, 2 out]
                        n150 = Index Array(array=w307, index=w306) -> (element=w305:string)
                        n151 = call "Tree_SetText_at_specified_Tag.vi"("New String IN"=w303, "Tag (whose string to be edited)"=w305, "Tree Refnum IN"=w304) -> ()  [unwired: 7 in, 2 out]
                      }
                      frame Enabled {
                      }
                    }
                  }
                  frame False {
                    # "Offset to factor in the outer FOR Loop"
                    # "Add new items to FGV"
                    n152 = for {
                      tunnel: w335 -> [w353] mode=indexing
                      tunnel: [w356] -> w334 mode=concatenating
                      n153 = call "Create Preset commands From Position Position-Power Row.vi"("Create SlowZ commands_Enum"=Create_Preset_commands_ENUM."Slow.Z_Move.To.Pos", "Position-Power Row"=w353) -> ("concatenated string"=w352:string)  [unwired: 9 in]
                      n154 = call "Create Preset commands From Position Position-Power Row.vi"("Create SlowZ commands_Enum"=Create_Preset_commands_ENUM."Slow.Z_Laser.Power", "Position-Power Row"=w353) -> ("concatenated string"=w351:string)  [unwired: 9 in]
                      n155 = Build Array(w352, w351, "Record()" ("Variable Name in")) -> (w356:string[])
                    }
                    n156 = Array Size(array=w334) -> (size(s)=w333:i32)
                    n157 = Multiply(x=w333, y=w332) -> (x*y=w331:i32)
                    n158 = for {
                      tunnel: w334 -> [w338] mode=indexing
                      tunnel: [w344] -> w336
                      tunnel: w337 -> [w345]
                      tunnel: w331 -> [w342]
                      tunnel: w330 -> [w340]
                      tunnel: w329 -> [w339]
                      i -> [w346]
                      n159 = Add(x=w346, y=w345) -> (x+y=w343:i32)
                      n160 = Add(x=w343, y=w342) -> (x+y=w341:i32)
                      n161 = call "FGV_MacroCore.vi"("MacroFGV_Commands"=FGV_MacroCore_Commands."Insert Item", "Start Index"=w341, "Macro Command or Info (String)"=w338) -> ("Macro String Array"=w344:string[])  [unwired: 4 in, 4 out]
                      n162 = disable-structure shown="Disabled" {
                        disable-tunnel: w340 -> [w350 _]
                        disable-tunnel: w339 -> [w349 _]
                        disable-tunnel: w338 -> [w348 _]
                        frame Disabled {
                          n163 = call "Tree_AddItem.vi"("NEW String"=w348, "Tag at add position"=w350, "Tree Refnum"=w349) -> ()  [unwired: 6 in, 3 out]
                        }
                        frame Enabled {
                        }
                      }
                    }
                  }
                }
              }
            }
            frame "Z-Stack (Regular)" {
              w368 = "pos.pockels.cell.PMT.Data" ("Variable Name in")
              w375 = "interpol Z stack data" ("Variable Name in")
              # "Restore saved \ninterpol data"
              # "Restore saved \ninterpol data"
              n164 = call "GFG_core.vi"("Variable Name in"="frames.per.plane", "Variant in"=w361, "error in (no error)"=w365, "Action"=enum16{"Init", "Set", "Get", "Clear"}."Set") -> ("error out"=w362:errorcluster)  [unwired: 9 in, 6 out]
              n165 = call "Wait till all GFG events stop_for fixed duration.vi"("error in (no error)"=w362) -> ("error out"=w359:errorcluster)  [unwired: 10 in]
              n166 = call "calculate tiling positions.vi"("error in (no error)"=w359, "overlap percentage"=w358) -> ("Array 2 - for Zstack tiling use this"=w360:dbl[][][])  [unwired: 7 in, 2 out]
              n167 = call "GFG_core.vi"("Variable Name in"=w375) -> ("Variant Out"=w383:variant)  [unwired: 12 in, 6 out]
              n168 = Variant To Data(error in=w359, type=dbl[][] [] ("Interpolated Data"), Variant=w383) -> (data=w379:dbl[][], error out=w381:errorcluster)
              n169 = disable-structure shown="Disabled" {
                disable-tunnel: [w390 _] -> w369
                disable-tunnel: w368 -> [w389 _]
                frame Disabled {
                  n170 = call "GFG_core.vi"("Variable Name in"=w389, "Action"=enum16{"Init", "Set", "Get", "Clear"}."Get") -> ("Variant Out"=w391:variant)  [unwired: 11 in, 6 out]
                  n171 = Variant To Data(type=dbl[][] [] ("Interpolated Data"), Variant=w391) -> (data=w390:dbl[][], error out=w393:errorcluster)  [unwired: 1 in]
                  n172 = call "Clear Specific Errors.vi"("Error In"=w393, "Error number In"=91) -> ()  [unwired: 8 in, 2 out]
                }
                frame Enabled {
                }
              }
              n173 = call "Clear Specific Errors.vi"("Error In"=w381, "Error number In"=91) -> ("Error Out"=w378:errorcluster)  [unwired: 8 in, 1 out]
              n174 = Empty Array?(array=w360) -> (empty?=w384:bool)
              n175 = for {
                tunnel: w360 -> [w426] mode=indexing
                shift-right: [w429] -> w374
                shift-left: w379 -> [w429]
                tunnel: w378 -> [_]
                tunnel: w375 -> [w428]
                shift-right: [w408] -> _
                shift-left: w377 -> [w410]
                tunnel: [w412] -> w366
                tunnel: w373 -> [w414]
                tunnel: w372 -> [w415]
                tunnel: [w411] -> w371
                shift-right: [w399] -> w367
                shift-left: w369 -> [w399]
                # "Create and save a new \nZ.Stack setup file"
                n176 = Transpose 2D Array(2D array=w426) -> (transposed array=w396:dbl[][])
                n177 = call "GFG_core.vi"("Variable Name in"=w428, "Variant in"=w396, "Action"=enum16{"Init", "Set", "Get", "Clear"}."Set") -> ("error out"=w420:errorcluster)  [unwired: 10 in, 6 out]
                n178 = Index Array(array=w426, index (row)=0) -> (element=w407:dbl[])  [unwired: 1 in]
                n179 = call "Wait till all GFG events stop_for fixed duration.vi"("error in (no error)"=w420) -> ("error out"=w401:errorcluster)  [unwired: 10 in]
                n180 = Index Array(array=w407, index #1=0 ("index"), index #2=1 ("index")) -> (element #1=w403:dbl, element #2=w404:dbl)
                n181 = for {
                  tunnel: w399 -> [w454] mode=indexing
                  tunnel: w404 -> [w451]
                  tunnel: w403 -> [w450]
                  tunnel: [w449] -> w402 mode=indexing
                  n182 = Replace Array Subset(array=w454, new element #1=w450, index #1=0 ("index"), new element #2=w451, index #2=1 ("index")) -> (w449:dbl[])
                }
                n183 = call "Create Preset commands From Position Position-Power Row.vi"("Create SlowZ commands_Enum"=Create_Preset_commands_ENUM."Slow.Z_Move.To.Pos", "Position-Power Row"=w407) -> ("concatenated string"=w422:string)  [unwired: 9 in]
                n184 = disable-structure shown="Enabled" {
                  disable-tunnel: w402 -> [w445 _]
                  disable-tunnel: w401 -> [w444 w448]
                  disable-tunnel: [w442 w448] -> w400
                  frame Disabled {
                    n185 = call "GFG_core.vi"("Variable Name in"="pos.pockels.cell.PMT.Data", "Variant in"=w445, "error in (no error)"=w444, "Action"=enum16{"Init", "Set", "Get", "Clear"}."Set") -> ("error out"=w443:errorcluster)  [unwired: 9 in, 6 out]
                    n186 = call "Wait till all GFG events stop_for fixed duration.vi"("error in (no error)"=w443) -> ("error out"=w442:errorcluster)  [unwired: 10 in]
                  }
                  frame Enabled {
                  }
                }
                n187 = call "FGV_MacroCore.vi"("Final Index"=w410, "MacroFGV_Commands"=FGV_MacroCore_Commands."Insert Item", "Error In"=w400, "Start Index"=w410, "Macro Command or Info (String)"=w422) -> ("Error Out"=w397:errorcluster, "Macro String Array"=w419:string[])  [unwired: 2 in, 3 out]
                n188 = Index Array(array=w419, index=w410) -> (element=w418:string)
                n189 = disable-structure shown="Disabled" {
                  disable-tunnel: w418 -> [w440 _]
                  disable-tunnel: [w439 w441] -> w417
                  disable-tunnel: w415 -> [w438 _]
                  disable-tunnel: w414 -> [w437 _]
                  disable-tunnel: w397 -> [w436 _]
                  disable-tunnel: w397 -> [_ w441]
                  frame Disabled {
                    n190 = call "Tree_AddItem.vi"("Error In"=w436, "NEW String"=w440, "Tag at add position"=w438, "Tree Refnum"=w437) -> ("Error Out"=w439:errorcluster)  [unwired: 5 in, 2 out]
                  }
                  frame Enabled {
                  }
                }
                n191 = Increment(x=w410) -> (x+1=w409:i32)
                n192 = call "FGV_MacroCore.vi"("Final Index"=w409, "MacroFGV_Commands"=FGV_MacroCore_Commands."Insert Item", "Error In"=w417, "Start Index"=w409, "Macro Command or Info (String)"="Z.Stack" ("concatenated string")) -> ("Error Out"=w413:errorcluster, "Macro String Array"=w411:string[])  [unwired: 2 in, 3 out]
                n193 = Index Array(array=w411, index=w409) -> (element=w416:string)
                n194 = disable-structure shown="Disabled" {
                  disable-tunnel: w416 -> [w434 _]
                  disable-tunnel: w415 -> [w433 _]
                  disable-tunnel: w414 -> [w432 _]
                  disable-tunnel: w413 -> [w431 w435]
                  disable-tunnel: [w430 w435] -> w412
                  frame Disabled {
                    n195 = call "Tree_AddItem.vi"("Error In"=w431, "NEW String"=w434, "Tag at add position"=w433, "Tree Refnum"=w432) -> ("Error Out"=w430:errorcluster)  [unwired: 5 in, 2 out]
                  }
                  frame Enabled {
                  }
                }
                n196 = Increment(x=w409) -> (x+1=w408:i32)
              }
              n197 = disable-structure shown="Disabled" {
                disable-tunnel: w368 -> [w387 _]
                disable-tunnel: w367 -> [w386 _]
                disable-tunnel: w366 -> [w385 _]
                frame Disabled {
                  n198 = call "GFG_core.vi"("Variable Name in"=w387, "Variant in"=w386, "error in (no error)"=w385, "Action"=enum16{"Init", "Set", "Get", "Clear"}."Set") -> ()  [unwired: 9 in, 7 out]
                }
                frame Enabled {
                }
              }
              n199 = call "GFG_core.vi"("Variable Name in"=w375, "Variant in"=w374, "error in (no error)"=w366, "Action"=enum16{"Init", "Set", "Get", "Clear"}."Set") -> ()  [unwired: 9 in, 7 out]
            }
            frame "Fast Z (Piezo)" {
              w466 = "pos.pockels.cell.PMT.Data" ("Variable Name in")
              w479 = "interpol Z stack data" ("Variable Name in")
              # "Restore saved \ninterpol data"
              # "Restore saved \ninterpol data"
              n200 = call "GFG_core.vi"("Variable Name in"="frames.per.plane", "Variant in"=w459, "error in (no error)"=w460, "Action"=enum16{"Init", "Set", "Get", "Clear"}."Set") -> ("error out"=w461:errorcluster)  [unwired: 9 in, 6 out]
              n201 = call "Wait till all GFG events stop_for fixed duration.vi"("error in (no error)"=w461) -> ("error out"=w458:errorcluster)  [unwired: 10 in]
              n202 = call "calculate tiling positions.vi"("error in (no error)"=w458, "overlap percentage"=w457) -> ("error out 2"=w455:errorcluster, "Array 2 - for Zstack tiling use this"=w456:dbl[][][])  [unwired: 7 in, 1 out]
              n203 = call "GFG_core.vi"("Variable Name in"=w466, "Action"=enum16{"Init", "Set", "Get", "Clear"}."Get") -> ("Variant Out"=w469:variant)  [unwired: 11 in, 6 out]
              n204 = call "GFG_core.vi"("Variable Name in"=w479) -> ("Variant Out"=w487:variant)  [unwired: 12 in, 6 out]
              n205 = Variant To Data(type=dbl[][] [] ("Interpolated Data"), Variant=w469) -> (data=w468:dbl[][], error out=w471:errorcluster)  [unwired: 1 in]
              n206 = Variant To Data(error in=w455, type=dbl[][] [] ("Interpolated Data"), Variant=w487) -> (data=w483:dbl[][], error out=w485:errorcluster)
              n207 = call "Clear Specific Errors.vi"("Error In"=w471, "Error number In"=91) -> ()  [unwired: 8 in, 2 out]
              n208 = call "Clear Specific Errors.vi"("Error In"=w485, "Error number In"=91) -> ("Error Out"=w482:errorcluster)  [unwired: 8 in, 1 out]
              n209 = for {
                tunnel: w456 -> [w520] mode=indexing
                shift-right: [w523] -> w478
                shift-left: w483 -> [w523]
                tunnel: w482 -> [_]
                tunnel: w479 -> [w522]
                shift-right: [w501] -> _
                shift-left: w481 -> [w503]
                tunnel: [w506] -> w464
                tunnel: w477 -> [w508]
                tunnel: w476 -> [w509]
                tunnel: [w505] -> w475
                shift-right: [w489] -> w465
                shift-left: w468 -> [w489]
                # "Create and save a new \nZ.Stack setup file"
                n210 = call "GFG_core.vi"("Variable Name in"=w522, "Variant in"=w520, "Action"=enum16{"Init", "Set", "Get", "Clear"}."Set") -> ("error out"=w514:errorcluster)  [unwired: 10 in, 6 out]
                n211 = Index Array(array=w520, index (row)=0) -> (element=w500:dbl[])  [unwired: 1 in]
                n212 = call "Wait till all GFG events stop_for fixed duration.vi"("error in (no error)"=w514) -> ("error out"=w492:errorcluster)  [unwired: 10 in]
                n213 = Index Array(array=w500, index #1=0 ("index"), index #2=1 ("index")) -> (element #1=w496:dbl, element #2=w497:dbl)
                n214 = for {
                  tunnel: w489 -> [w541] mode=indexing
                  tunnel: w497 -> [w538]
                  tunnel: w496 -> [w537]
                  tunnel: [w536] -> w493 mode=indexing
                  n215 = Replace Array Subset(array=w541, new element #1=w537, index #1=0 ("index"), new element #2=w538, index #2=1 ("index")) -> (w536:dbl[])
                }
                n216 = call "Create Preset commands From Position Position-Power Row.vi"("Create SlowZ commands_Enum"=Create_Preset_commands_ENUM."Slow.Z_Move.To.Pos", "Position-Power Row"=w500) -> ("concatenated string"=w516:string)  [unwired: 9 in]
                n217 = call "GFG_core.vi"("Variable Name in"="pos.pockels.cell.PMT.Data", "Variant in"=w493, "error in (no error)"=w492, "Action"=enum16{"Init", "Set", "Get", "Clear"}."Set") -> ("error out"=w491:errorcluster)  [unwired: 9 in, 6 out]
                n218 = call "Wait till all GFG events stop_for fixed duration.vi"("error in (no error)"=w491) -> ("error out"=w490:errorcluster)  [unwired: 10 in]
                n219 = call "FGV_MacroCore.vi"("Final Index"=w503, "MacroFGV_Commands"=FGV_MacroCore_Commands."Insert Item", "Error In"=w490, "Start Index"=w503, "Macro Command or Info (String)"=w516) -> ("Error Out"=w504:errorcluster, "Macro String Array"=w513:string[])  [unwired: 2 in, 3 out]
                n220 = Index Array(array=w513, index=w503) -> (element=w512:string)
                n221 = disable-structure shown="Enabled" {
                  disable-tunnel: w512 -> [w534 _]
                  disable-tunnel: [w533 w535] -> w511
                  disable-tunnel: w509 -> [w532 _]
                  disable-tunnel: w508 -> [w531 _]
                  disable-tunnel: w504 -> [w530 w535]
                  frame Disabled {
                    n222 = call "Tree_AddItem.vi"("Error In"=w530, "NEW String"=w534, "Tag at add position"=w532, "Tree Refnum"=w531) -> ("Error Out"=w533:errorcluster)  [unwired: 5 in, 2 out]
                  }
                  frame Enabled {
                  }
                }
                n223 = Increment(x=w503) -> (x+1=w502:i32)
                n224 = call "FGV_MacroCore.vi"("Final Index"=w502, "MacroFGV_Commands"=FGV_MacroCore_Commands."Insert Item", "Error In"=w511, "Start Index"=w502, "Macro Command or Info (String)"="Fast.Z" ("concatenated string")) -> ("Error Out"=w507:errorcluster, "Macro String Array"=w505:string[])  [unwired: 2 in, 3 out]
                n225 = Index Array(array=w505, index=w502) -> (element=w510:string)
                n226 = disable-structure shown="Disabled" {
                  disable-tunnel: w510 -> [w529 _]
                  disable-tunnel: w509 -> [w528 _]
                  disable-tunnel: w508 -> [w527 _]
                  disable-tunnel: w507 -> [w526 _]
                  disable-tunnel: [w525 _] -> w506
                  frame Disabled {
                    n227 = call "Tree_AddItem.vi"("Error In"=w526, "NEW String"=w529, "Tag at add position"=w528, "Tree Refnum"=w527) -> ("Error Out"=w525:errorcluster)  [unwired: 5 in, 2 out]
                  }
                  frame Enabled {
                  }
                }
                n228 = Increment(x=w502) -> (x+1=w501:i32)
              }
              n229 = Empty Array?(array=w456) -> (empty?=w488:bool)
              n230 = call "GFG_core.vi"("Variable Name in"=w466, "Variant in"=w465, "error in (no error)"=w464, "Action"=enum16{"Init", "Set", "Get", "Clear"}."Set") -> ()  [unwired: 9 in, 7 out]
              n231 = call "GFG_core.vi"("Variable Name in"=w479, "Variant in"=w478, "error in (no error)"=w464, "Action"=enum16{"Init", "Set", "Get", "Clear"}."Set") -> ()  [unwired: 9 in, 7 out]
            }
          }
          n232 = flat-sequence {
            tunnel: w178 -> [w189]
            tunnel: w176 -> [w185]
            tunnel: w175 -> [_]
            frame #0 {
              n233 = invoke class="Tree" method="Edit Tree Items.Delete"(reference=w189, "Delete Children"=TRUE ("Delete Children?")) -> (reference out=w187:refnum<vi>, error out=w186:errorcluster)  [unwired: 3 in, 3 out]
              n234 = disable-structure shown="Enabled" {
                disable-tunnel: w187 -> [w192 _]
                disable-tunnel: w186 -> [w191 _]
                disable-tunnel: w185 -> [w190 _]
                frame Enabled {
                  n235 = invoke class="Tree" method="Edit Tree Items.Add Multiple Items to End"(reference=w192, error in=w191, "Items"=w190) -> ()  [unwired: 1 in, 4 out]
                }
                frame Disabled {
                }
              }
            }
          }
          n236 = call "FGV_MacroCore.vi"("MacroFGV_Commands"=FGV_MacroCore_Commands."Get Array", "Error In"=w172) -> ("Macro String Array"=w173:string[])  [unwired: 5 in, 4 out]
          n237 = for {
            tunnel: w173 -> [w194] mode=indexing
            tunnel: [w193] -> w176 mode=indexing
            n238 = Bundle By Name(cluster=T6 {"Left Cell String"="", "Child Text"=[], "Child Tag"="", "Item Indent"=0, "Child Only?"=FALSE, "Glyph Index"=0} ("Item"), "Left Cell String"=w194) -> (w193:T6)
          }
        }
        frame #1 {
          n239 = call <vilib>:"Unset Busy.vi"() -> ()  [unwired: 11 in, 1 out]
        }
      }
      n240 = Add(x=w154, y=2) -> (x+y=w159:i32)
    }
    frame True {
    }
  }
  n241 = flat-sequence {
    tunnel: w36 -> [w584]
    tunnel: w30 -> [w583]
    tunnel: w29 -> [w582]
    tunnel: w27 -> [w581]
    tunnel: w2 -> [w579]
    frame #0 {
      n242 = Not(x=w579) -> (.not. x?=w578:bool)
      n243 = call "bring vi to front.vi"("VI Name"="MacroGUI_MD.vi") -> ()  [unwired: 11 in]
      n244 = case shown="True" w578 {
        frame False {
        }
        frame True {
          n245 = call-poly "GFGpolyGet.vi"("Variable Name in"="Cancel" ("VI Name")) -> ("output cluster"=w587:T9)  [unwired: 9 in, 1 out]
          n246 = Unbundle By Name(w587) -> ("BooleanRef"=w586:refnum<vi>)
          n247 = property class="Bool"(reference=w586, "Val(Sgnl)"=TRUE ("empty?")) -> ()  [unwired: 1 in, 2 out]
        }
      }
      "Index of 2DFrame.Scan" <- w584
      "Updated Macro String Array" <- w583
      "Empty Array/Cancelled?" <- w582
      "Skip configure 2D settings?" <- w581
    }
  }
  "error out" <- "error in (no error)"
